vi "Dashboard Main.vi"() -> ()   [LabVIEW 2012]
uses:
  <vilib>/event_ctls.llb/eventvkey.ctl
  <vilib>/Utility/config.llb/Read Key (String).vi
  <vilib>/Utility/config.llb/Read Key (I32).vi
  <vilib>/Utility/config.llb/Write Key (String).vi
  <vilib>/Utility/config.llb/Write Key (I32).vi
  <vilib>/Utility/config.llb/NI_LVConfig.lvlib
panel:
  out "Battery Value":dbl(slide) scale=0.0..14.0 scale format="%#_2e"
  out "Battery":sgl(graph)
  in  "Camera Settings":T1={"Frate Rate"=30, "Compression"=30, "Size"=1} {"Frate Rate" scale=1.0..30.0; "Size" items=["640x480", "320x240", "160x120"]}
  out "Mode":T2(ring)=enum."Auto Disabled"
  out "Camera IP":string
  out "JS1 Z":dbl(slide) scale=-1.0..1.0 scale format="%#_2e"
  out "JS2 Z":dbl(slide) scale=-1.0..1.0 scale format="%#_2e"
  out "Joystick 1":cluster{"X":dbl, "Y":dbl}[](graph)
  out "Joystick 2":cluster{"X":dbl, "Y":dbl}[](graph)
  out "JS Buttons 1":T3
  out "JS Buttons 2":T3
  out "MotorSlide4":dbl(slide) scale=-1.0..1.0 scale format="%#_2e"
  out "MotorSlide3":dbl(slide) scale=-1.0..1.0 scale format="%#_2e"
  out "MotorSlide2":dbl(slide) scale=-1.0..1.0 scale format="%#_2e"
  in  "MotorName3":string="Front Left"
  in  "MotorName4":string="Front Right"
  in  "MotorName1":string="Rear Left"
  in  "MotorName2":string="Rear Right"
  out "MotorChart4":dbl(graph)
  out "MotorChart3":dbl(graph)
  out "MotorChart2":dbl(graph)
  out "MotorSlide1":dbl(slide) scale=-1.0..1.0 scale format="%#_2e"
  out "MotorChart1":dbl(graph)
  out "Robot IP":string
  in  "Dashboard Tab":enum32{"Operation", "Test", "Checklist"}(tab)
  in  "Checkbox 2":bool
  in  "Checkbox 1":bool
  in  "Slider 1":dbl(slide) scale=0.0..100.0
  out "array of clusters":cluster{"vi reference":refnum<vi>}[](array[cluster])
  in  "Slider":dbl(slide) scale=0.0..100.0 scale format="%#_3g"
  in  "On/Off":bool caption="Solenoid"
  in  "Test Name":u16(ring) items=["Select the test to run...", "Example Test", "-------------------------------", "List of tests is built in robot code.", "Replace with your own automated tests."]
  in  "Test Tree":string(tree)
  in  "Motor":cluster{"Value":dbl, "Enable":bool} {"Value" scale=-1.0..1.0 scale format="%#_3g"}
  out "Progress":T4 {"Test Progress" scale=0.0..100.0}
  in  "Rev/Fwd":cluster{"Forward":bool, "Reverse":bool}
  in  "Ring":u16(ring) items=["Auto", "Fixed indoor", "Fixed outdoor 1", "Fixed outdoor 2", "Fixed fluorescent 1", "Fixed fluorescent 2", "Hold current"]
  in  "Listbox":i32(listbox)
  in  "Viewer":T5(tab)
  out "Mbps":dbl format="%#.1g"
  in  "Enable":bool
  in  "DB Camera Config":bool
  out "Mbps":bool
  out "fps":dbl format="%#.1g"
  out "Image Error Message":string="Timeout in Camera Communications"
  out "Camera Image":T6(plugin-control)
  out "Buttons 1":cluster{"1":bool, "2":bool, "3":bool}
  out "Kinect 1":cluster{"X":dbl, "Y":dbl, "Z":dbl} {"X" scale=1.0..-1.0; "Y" scale=1.0..-1.0; "Z" scale=1.0..-1.0}
  out "Buttons 2":cluster{"1":bool, "2":bool, "3":bool}
  out "Kinect 2":cluster{"X":dbl, "Y":dbl, "Z":dbl} {"X" scale=1.0..-1.0; "Y" scale=1.0..-1.0; "Z" scale=1.0..-1.0}
  out "Version":string
  out "Skeleton Picture":picture
  out "Players":i8
  out "Tree":string(tree)
  # "Drive & Motors"
  # "Robot IP:"
  # "Customize by placing controls and indicators here and name to match\nDashboard Variables on robot."
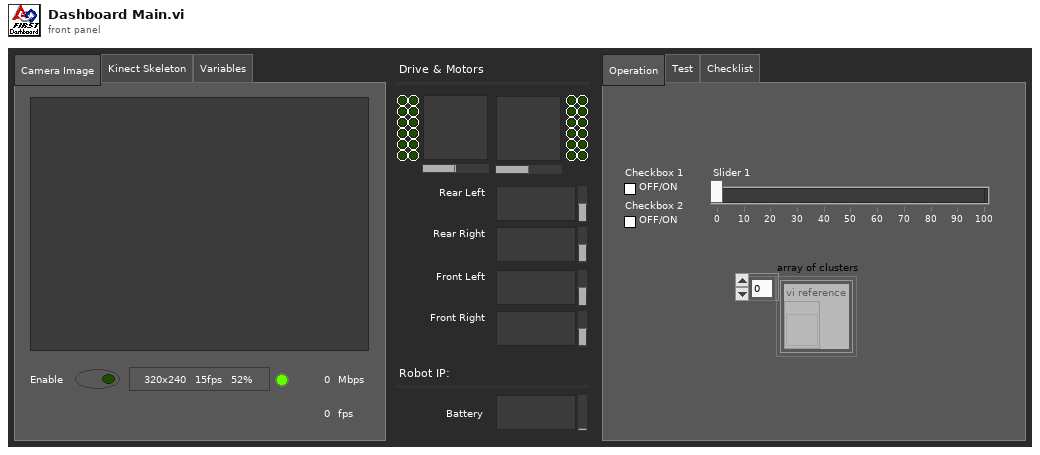
[diagram p1: front panel]
types:
  T1 = cluster{"Frate Rate":i32, "Compression":i32, "Size":u16}
  T2 = enum8{"Tele-Op Disabled", "Tele-Op Enabled", "Auto Disabled", "Auto Enabled", "Test Disabled", "Test Enabled", ""}
  T3 = cluster{bool, bool, bool, bool, bool, bool, bool, bool, bool, bool, bool, bool}
  T4 = cluster{"Test Progress":u8, "Test Progress Text":string}
  T5 = enum32{"Camera Image", "Kinect Skeleton", "Variables"}
  T6 = typedef "IMAQ Image.ctl" = refnum<image>
  T7 = typedef "Image Type" = u32
  T8 = typedef "LVBoundsTypeDef.ctl" = cluster{"Width":u32, "Height":u32}
  T9 = typedef "SkeletonTrackState.ctl" = enum32{"NotTracked", "PositionOnly", "Tracked"}
  T10 = cluster{"TrackingState":u8[], "Position":cluster{"x":sgl, "y":sgl, "z":sgl}, cluster{"x":sgl, "y":sgl, "z":sgl, sgl}[], "TrackState":T9}
  T11 = cluster{cluster{"ScaledToPercentRange":dbl, "ScaledToPercentRange":dbl, "ScaledToPercentRange":dbl}, cluster{bool, bool, bool}}[]
  T12 = cluster{cluster{"ScaledToPercentRange":dbl, "ScaledToPercentRange":dbl, "ScaledToPercentRange":dbl}, cluster{bool, bool, bool}}
  T13 = cluster{"ScaledToPercentRange":dbl, "ScaledToPercentRange":dbl, "ScaledToPercentRange":dbl}
  T14 = typedef "LVRectTypeDef.ctl" = cluster{"Left":i16, "Top":i16, "Right":i16, "Bottom":i16}
  T15 = cluster{"Competition mode":bool, "Robot Link":bool, "Autonomous":bool, "Enabled":bool, "E-Stop":bool, "Simulated":bool, "TestMode":bool, "Docked Window":bool}
  T16 = cluster{"Boolean Array[0]":bool, "Boolean Array[1]":bool, "Boolean Array[2]":bool, "Boolean Array[3]":bool, "Boolean Array[4]":bool, "Boolean Array[5]":bool, "Boolean Array[6]":bool, "Boolean Array[7]":bool, "Boolean Array[8]":bool, "Boolean Array[9]":bool, "Boolean Array[10]":bool, "Boolean Array[11]":bool}
  T17 = typedef "NI_LVConfig.lvlib/Config Data RefNum.ctl" = refnum<k1>
  T18 = typedef "eventvkey.ctl" = enum16{"ASCII", "Enter", "Return", "Shift", "Ctrl", "Alt", "Cmd", "Opt", "Caps", "NumLock", "Clear", "Break", "Up", "Down", "Left", "Right", "Insert", "Delete", "Home", "End", "PageUp", "PageDown", "Escape", "Help", "Pause", "ScrollLock", "F1", "F2", "F3", "F4", "F5", "F6", "F7", "F8", "F9", "F10", "F11", "F12", "F13", "F14", "F15", "F16", "F17", "F18", "F19", "F20", "F21", "F22", "F23", "F24", "Play", "VolumeUp", "VolumeDown", "Mute", "Two Byte Char"}
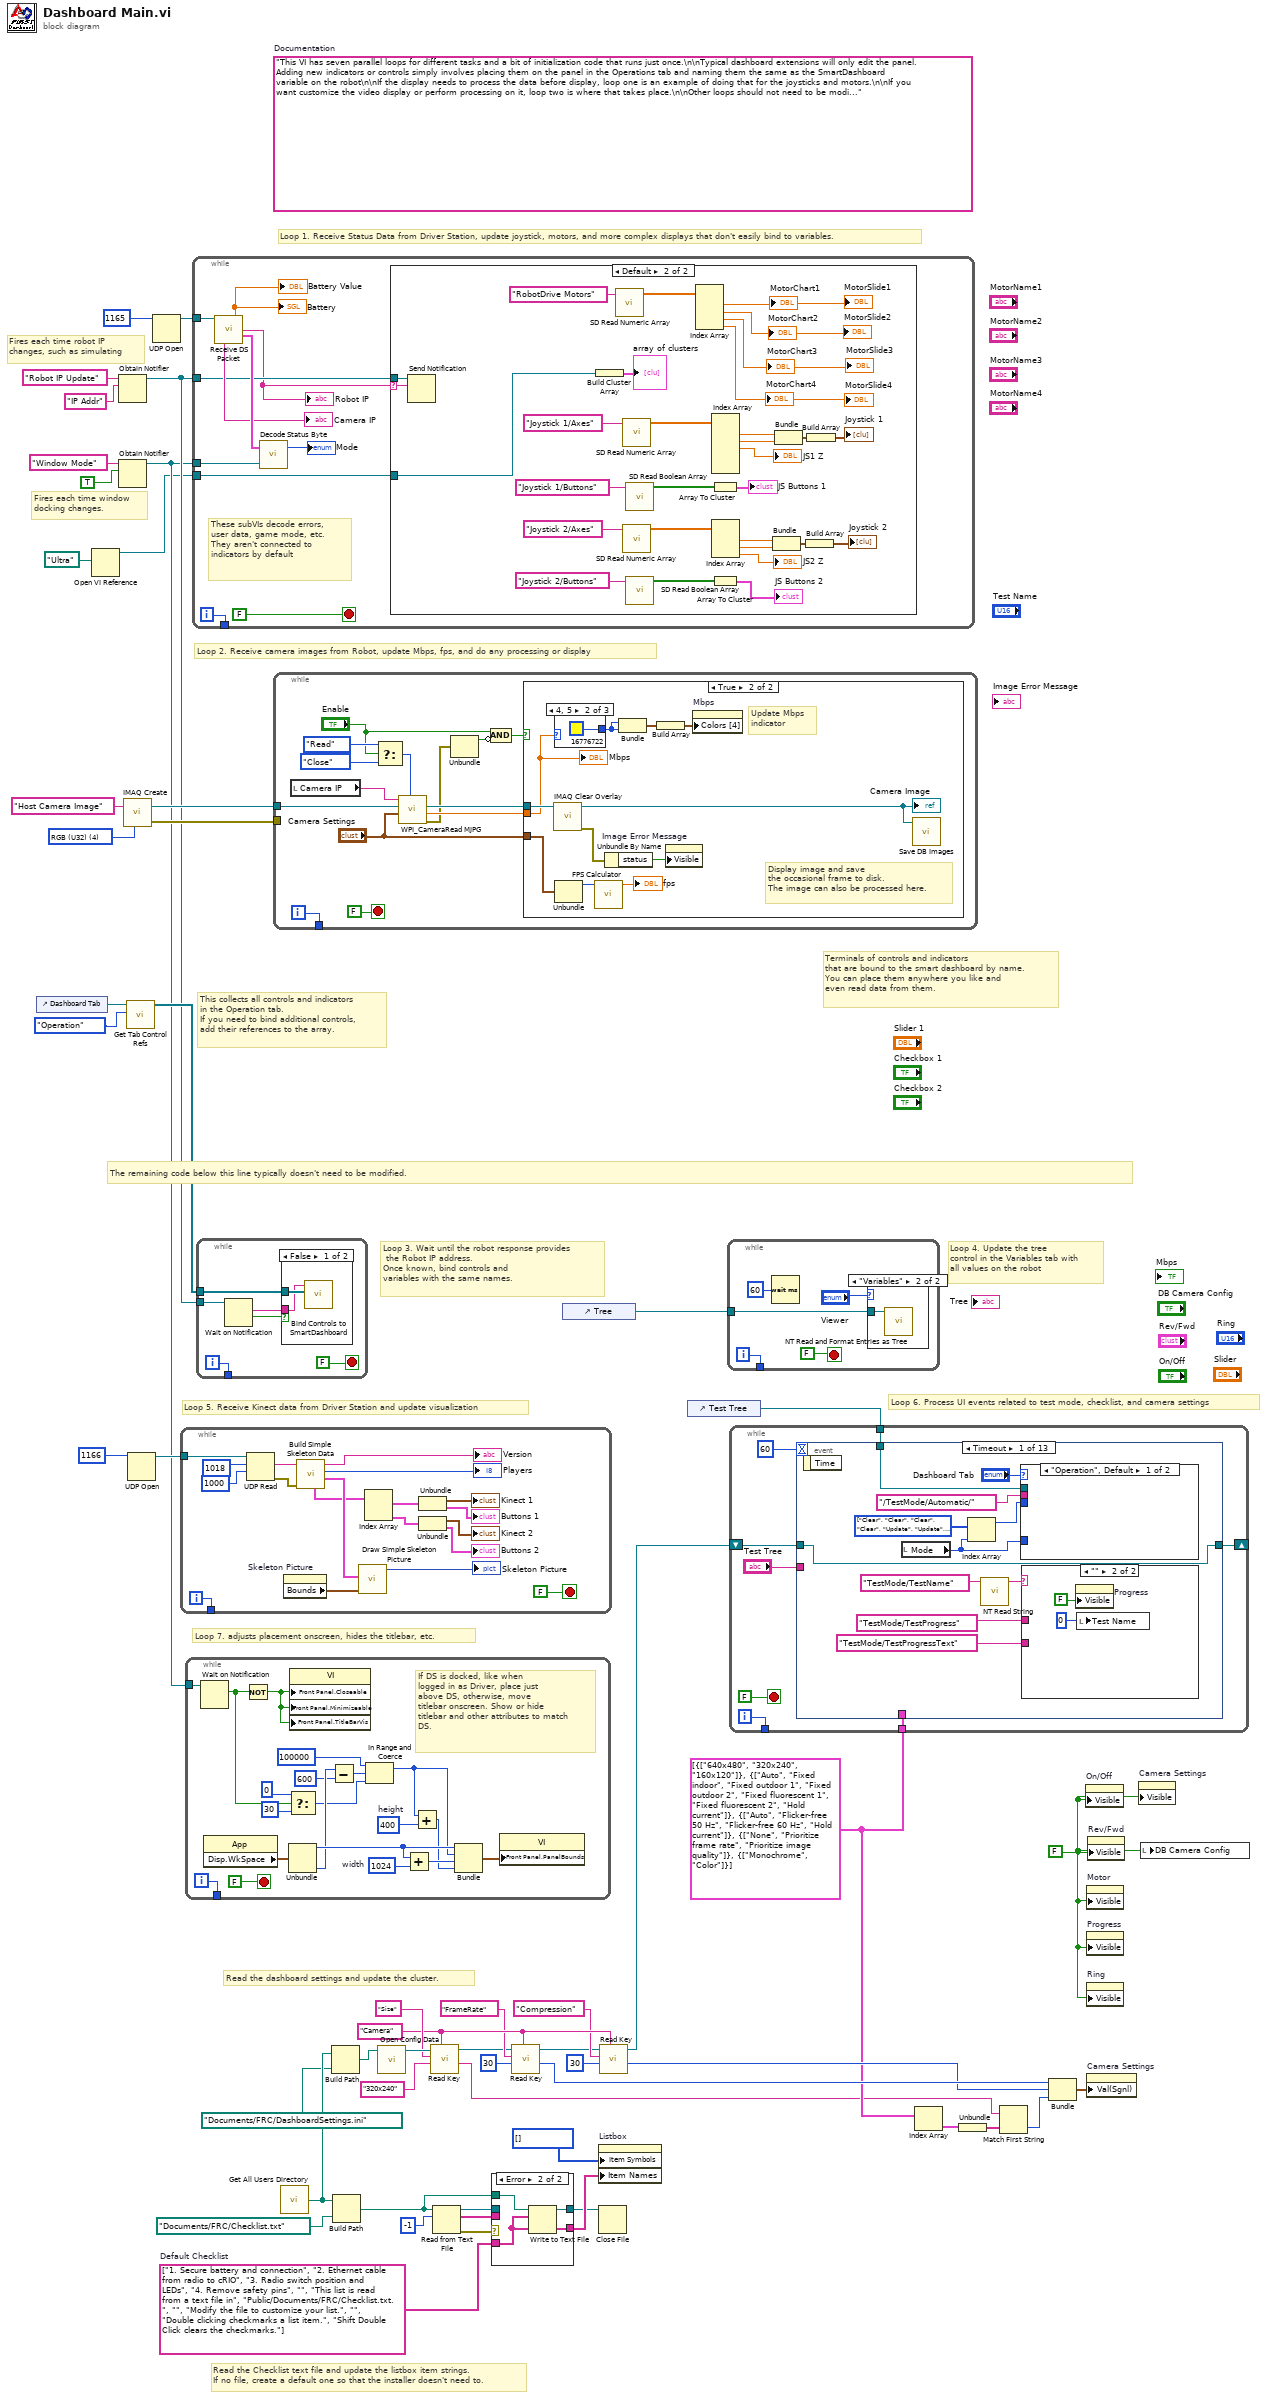
[diagram p0: block diagram]
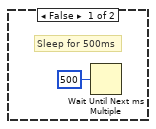
[diagram p3: hidden frame]
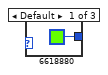
[diagram p4: hidden frame]
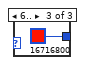
[diagram p5: hidden frame]
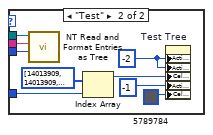
[diagram p7: hidden frame]
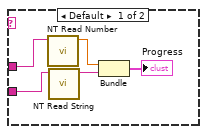
[diagram p8: hidden frame]
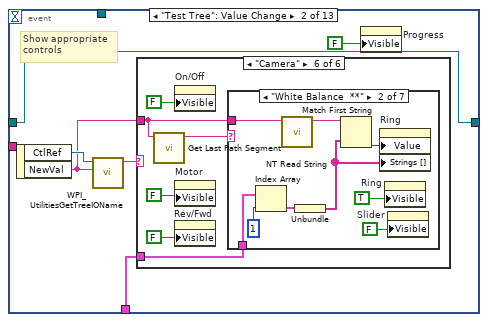
[diagram p9: hidden frame]
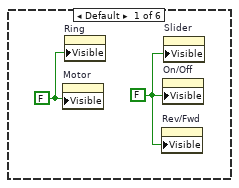
[diagram p10: hidden frame]
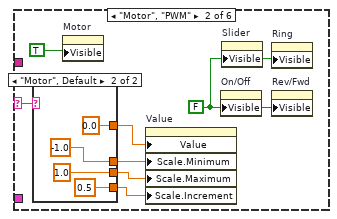
[diagram p11: hidden frame]
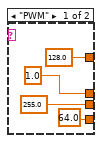
[diagram p12: hidden frame]
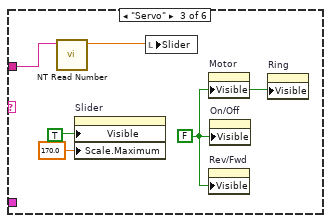
[diagram p13: hidden frame]
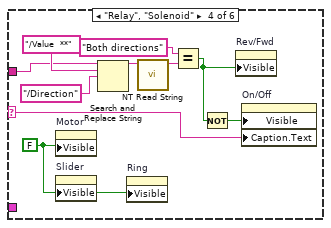
[diagram p14: hidden frame]
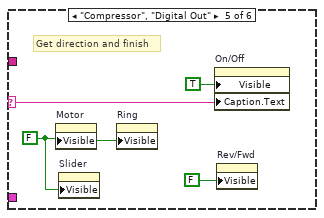
[diagram p15: hidden frame]
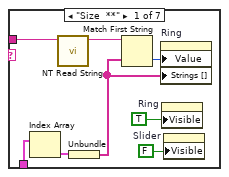
[diagram p16: hidden frame]
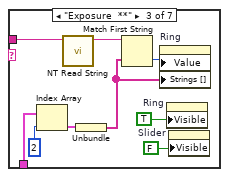
[diagram p17: hidden frame]
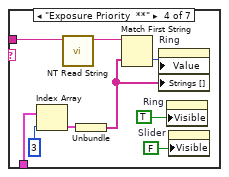
[diagram p18: hidden frame]
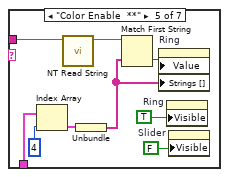
[diagram p19: hidden frame]
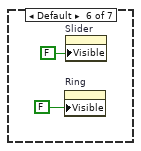
[diagram p20: hidden frame]
diagram:
  w23 = "Camera"
  w15 = cluster{string[]}[] [{["640x480", "320x240", "160x120"]}, {["Auto", "Fixed indoor", "Fixed outdoor 1", "Fixed outdoor 2", "Fixed fluorescent 1", "Fixed fluorescent 2", "Hold current"]}, {["Auto", "Flicker-free 50 Hz", "Flicker-free 60 Hz", "Hold current"]}, {["None", "Prioritize frame rate", "Prioritize image quality"]}, {["Monochrome", "Color"]}]
  w31 = string[] ["1. Secure battery and connection", "2. Ethernet cable from radio to cRIO", "3. Radio switch position and LEDs", "4. Remove safety pins", "", "This list is read from a text file in", "Public/Documents/FRC/Checklist.txt.", "", "Modify the file to customize your list.", "", "Double clicking checkmarks a list item.", "Shift Double Click clears the checkmarks."]  # Default Checklist
  w29 = FALSE ("Visible")
  (unwired) "This VI has seven parallel loops for different tasks and a bit of initialization code that runs just once.\n\nTypical dashboard extensions will only edit the panel. Adding new indicators or controls simply involves placing them on the panel in the Operations tab and naming them the same as the SmartDashboard variable on the robot\n\nIf the display needs to process the data before display, loop one is an example of doing that for the joysticks and motors.\n\nIf you want customize the video display or perform processing on it, loop two is where that takes place.\n\nOther loops should not need to be modified. They are pretty standard, and document the task they perform."  # Documentation
  w52 = T7 4 items=["Grayscale (U8)", "Grayscale (I16)", "Grayscale (SGL)", "Complex (CSG)", "RGB (U32)", "HSL (U32)", "RGB (U64)"] ("Image Type")
  # "Fires each time robot IP\nchanges, such as simulating"
  # "Fires each time window\ndocking changes."
  # "Read the Checklist text file and update the listbox item strings.\nIf no file, create a default one so that the installer doesn't need to."
  # "This collects all controls and indicators\nin the Operation tab.\nIf you need to bind additional controls,\nadd their references to the array."
  # "The remaining code below this line typically doesn't need to be modified."
  # "Loop 6. Process UI events related to test mode, checklist, and camera settings"
  # "Read the dashboard settings and update the cluster."
  # "Terminals of controls and indicators\nthat are bound to the smart dashboard by name.\nYou can place them anywhere you like and\neven read data from them."
  # "Loop 4. Update the tree\ncontrol in the Variables tab with\nall values on the robot"
  # "Loop 3. Wait until the robot response provides\n the Robot IP address.\nOnce known, bind controls and\nvariables with the same names."
  # "Loop 5. Receive Kinect data from Driver Station and update visualization"
  # "Loop 7. adjusts placement onscreen, hides the titlebar, etc."
  # "Loop 1. Receive Status Data from Driver Station, update joystick, motors, and more complex displays that don't easily bind to variables."
  # "Loop 2. Receive camera images from Robot, update Mbps, fps, and do any processing or display"
  n1 = control-ref of="Dashboard Tab"() -> (w45:refnum<vi>)
  n2 = Open VI Reference(vi path=path "Ultra") -> (vi reference=w1:refnum<vi>)  [unwired: 5 in, 1 out]
  n3 = Obtain Notifier(name (unnamed)="Robot IP Update", notification data type="IP Addr" ("name (unnamed)")) -> (notifier out=w42:refnum<notifier>)  [unwired: 2 in, 2 out]
  n4 = Obtain Notifier(name (unnamed)="Window Mode", notification data type=TRUE) -> (notifier out=w35:refnum<notifier>)  [unwired: 2 in, 2 out]
  n5 = call "IMAQ Create"("Image Name"="Host Camera Image", "Image Type"=w52) -> ("New Image"=w50:T6, "error out"=w49:errorcluster)  [unwired: 2 in, 1 out]
  n6 = call <vilib>:"Get Tab Control Refs.vi"("Page Index"=enum32{"Operation", "Test"}."Operation" ("Dashboard Tab"), "TabControl in"=w45) -> ("ControlsOnPage"=w46:refnum<vi>[])  [unwired: 9 in]
  n7 = UDP Open(11:u16 1166 ("port")) -> (port=w47:refnum<k16>)  [unwired: 2 in, 4 out]
  n8 = UDP Open(11:u16 1165 ("port")) -> (port=w53:refnum<k16>)  [unwired: 2 in, 4 out]
  n9 = while {
    tunnel: w47 -> [w71]
    tunnel: [w56] -> _
    i -> [w56]
    stop <- FALSE stop-if-true
    n10 = UDP Read(connection ID=w71, max size (548)=1018 ("bytes to read"), timeout ms (25000)=1000) -> (data out=w65:string, error out=w55:errorcluster)  [unwired: 1 in, 3 out]
    n11 = property on="Skeleton Picture" class="Pict"() -> ("Bounds"=w67:T8)  [unwired: 2 in, 2 out]
    n12 = call "Build Simple Skeleton Data.vi"("error in (no error)"=w55, "data in"=w65) -> ("Skeleton Data"=w66:T10, "NumPlayers"=→"Players":i8, "Version String"=→"Version":string, "Simple Joystick Info"=w63:T11)  [unwired: 5 in, 1 out]
    n13 = call "Draw Simple Skeleton Picture.vi"("Bounds"=w67, "Simple Skeleton"=w66) -> ("new picture out"=→"Skeleton Picture":picture)  [unwired: 9 in]
    n14 = Index Array(array=w63) -> (element #1=w62:T12, element #2=w61:T12)  [unwired: 2 in]
    n15 = Unbundle(w62) -> (→"Kinect 1":T13, →"Buttons 1":cluster{bool, bool, bool})
    n16 = Unbundle(w61) -> (→"Kinect 2":T13, →"Buttons 2":cluster{bool, bool, bool})
  }
  n17 = while {
    tunnel: w35 -> [w92]
    tunnel: [w90] -> _
    i -> [w90]
    stop <- FALSE stop-if-true
    w82 = 1024  # width
    w85 = 400  # height
    # "If DS is docked, like when\nlogged in as Driver, place just\nabove DS, otherwise, move\ntitlebar onscreen. Show or hide\ntitlebar and other attributes to match\nDS."
    n18 = Wait on Notification(notifier=w92) -> (notification=w77:bool)  [unwired: 3 in, 3 out]
    n19 = property class="App"() -> ("Disp.WkSpace"=w88:T14)  [unwired: 2 in, 2 out]
    n20 = Not(x=w77) -> (.not. x?=w91:bool)
    n21 = Unbundle(w88) -> ("Left"=w86:i16, "Bottom"=w83:i16)  [unwired: 2 out]
    n22 = Select(t=0, s=w77, f=30) -> (s? t:f=w76:i32)
    n23 = property class="VI"("Front Panel.Closeable"=w91, "Front Panel.Minimizeable"=w91, "Front Panel.TitleBarVis"=w91) -> ()  [unwired: 2 in, 2 out]
    n24 = Subtract(x=w83, y=600) -> (x-y=w80:i32)
    n25 = In Range and Coerce(upper limit=100000, x=w80, lower limit=w76) -> (coerced(x)=w74:i32)  [unwired: 1 out]
    n26 = Add(x=w86, y=w82) -> (x+y=w87:i32)
    n27 = Add(x=w74, y=w85) -> (x+y=w84:i32)
    n28 = Bundle("Left"=w86, w74, w87, w84) -> (w89:cluster{"Left":i16, i32, i32, i32})  [unwired: 1 out]
    n29 = property class="VI"("Front Panel.PanelBounds"=w89) -> ()  [unwired: 2 in, 2 out]
  }
  n30 = while {
    tunnel: w53 -> [w102]
    tunnel: w42 -> [w96]
    tunnel: w35 -> [w100]
    tunnel: [w97] -> _
    tunnel: w1 -> [w94]
    i -> [w97]
    stop <- FALSE stop-if-true
    # "These subVIs decode errors, user data, game mode, etc.\nThey aren't connected to indicators by default"
    n31 = call "Receive DS Packet.vi"("Recv Socket"=w102) -> ("Battery"=→"Battery" →"Battery Value":sgl, "Robot IP Address"=w95:string, "Status"=w103:T15, "Camera IP Address"=→"Camera IP":string)  [unwired: 1 in, 10 out]
    "Robot IP" <- w95
    n32 = call "Decode Status Byte.vi"("Window Mode Notifier"=w100, "Status"=w103) -> ("Mode"=→"Mode":T2)  [unwired: 1 out]
    n33 = case shown="Default" w95 {
      selector: w95 -> [_ w107]
      tunnel: w96 -> [_ w108]
      tunnel: w94 -> [_ w105]
      frame "0.0.0.0" {
        # "Robot not responding, don't poll the variables"
      }
      frame Default {
        n34 = Send Notification(notification=w107, notifier=w108) -> ()  [unwired: 1 in, 2 out]
        n35 = Build Cluster Array(w105) -> (→"array of clusters":cluster{"vi reference":refnum<vi>}[])
        n36 = call <vilib>:"SD Read Numeric Array.vi"("Name"="RobotDrive Motors") -> ("Numeric Array"=w131:dbl[])  [unwired: 8 in, 2 out]
        n37 = call <vilib>:"SD Read Numeric Array.vi"("Name"="Joystick 1/Axes") -> ("Numeric Array"=w124:dbl[])  [unwired: 8 in, 2 out]
        n38 = call <vilib>:"SD Read Numeric Array.vi"("Name"="Joystick 2/Axes") -> ("Numeric Array"=w118:dbl[])  [unwired: 8 in, 2 out]
        n39 = call <vilib>:"SD Read Boolean Array.vi"("Name"="Joystick 1/Buttons") -> ("Boolean Array"=w126:bool[])  [unwired: 8 in, 2 out]
        n40 = call <vilib>:"SD Read Boolean Array.vi"("Name"="Joystick 2/Buttons") -> ("Boolean Array"=w117:bool[])  [unwired: 8 in, 2 out]
        n41 = Index Array(array=w131) -> (element #1=→"MotorChart1" →"MotorSlide1":dbl, element #2=→"MotorSlide2" →"MotorChart2":dbl, element #3=→"MotorChart3" →"MotorSlide3":dbl, element #4=→"MotorChart4" →"MotorSlide4":dbl)  [unwired: 4 in]
        n42 = Array To Cluster(array=w126) -> (cluster=→"JS Buttons 1":T16)
        n43 = Array To Cluster(array=w117) -> (cluster=→"JS Buttons 2":T16)
        n44 = Index Array(array=w124) -> (element #1=w121:dbl, element #2=w122:dbl, element #3=→"JS1 Z":dbl)  [unwired: 6 in, 3 out]
        n45 = Index Array(array=w118) -> (element #1=w113:dbl, element #2=w112:dbl, element #3=→"JS2 Z":dbl)  [unwired: 3 in]
        n46 = Bundle("Numeric"=w113, "Numeric"=w112) -> (w114:cluster{"Numeric":dbl, "Numeric":dbl})  [unwired: 1 in]
        n47 = Bundle("Numeric"=w121, "Numeric"=w122) -> (w120:cluster{"Numeric":dbl, "Numeric":dbl})  [unwired: 1 in]
        n48 = Build Array(w114) -> (→"Joystick 2":cluster{"Numeric":dbl, "Numeric":dbl}[])
        n49 = Build Array(w120) -> (→"Joystick 1":cluster{"Numeric":dbl, "Numeric":dbl}[])
      }
    }
  }
  n50 = while {
    tunnel: w46 -> [w140]
    tunnel: w42 -> [w137]
    tunnel: [w135] -> _
    i -> [w135]
    stop <- FALSE stop-if-true
    n51 = Wait on Notification(notifier=w137) -> (notification=w136:string, timed out?=w138:bool)  [unwired: 3 in, 2 out]
    n52 = case shown="False" w138 {
      tunnel: w140 -> [w142 _]
      tunnel: w136 -> [w141 _]
      frame False {
        n53 = call <vilib>:"Bind Controls to SmartDashboard.vi"("Bound Control Refs"=w142, "Server IP Address"=w141) -> ()  [unwired: 10 in]
      }
      frame True {
      }
    }
  }
  n54 = while {
    tunnel: w50 -> [w152]
    tunnel: w49 -> [_]
    tunnel: [w155] -> _
    i -> [w155]
    stop <- FALSE stop-if-true
    n55 = local read "Camera IP"() -> (w154:string)
    n56 = Select(t=enum16{"Read", "Reopen", "Close"}."Read" ("Operation"), s="Enable", f=enum16{"Read", "Reopen", "Close"}."Close" ("Operation")) -> (s? t:f=w147:enum16{"Read", "Reopen", "Close"})
    n57 = call <vilib>:"WPI_CameraRead MJPG.vi"("Operation"=w147, "Camera Settings"="Camera Settings", "Image"=w152, "address"=w154) -> ("error out"=w146:errorcluster, "Bandwidth (kbps)"=w150:dbl, "Image Out"=w151:T6)  [unwired: 5 in]
    n58 = Unbundle(w146) -> ("status"=w144:bool)  [unwired: 2 out]
    n59 = Compound Arithmetic op=AND("Enable", invert w144) -> (w143:bool)
    n60 = case shown="True" w143 {
      tunnel: "Camera Settings" -> [_ w159]
      tunnel: w151 -> [_ w162]
      tunnel: w150 -> [_ w161]
      frame False {
        # "Sleep for 500ms"
        n61 = Wait Until Next ms Multiple(millisecond multiple=u32 500) -> ()  [unwired: 1 out]
      }
      frame True {
        # "Display image and save\nthe occasional frame to disk.\nThe image can also be processed here."
        # "Update Mbps\nindicator"
        n62 = call "IMAQ Clear Overlay"("Image"=w162) -> ("error out"=w167:errorcluster, "Image Out"=w166:T6)  [unwired: 2 in, 7 out]
        "Camera Image" <- w166
        n63 = case shown="4, 5" w161 {
          tunnel: [u32 6618880 ("Color Box") u32 16776722 ("Color Box") u32 16716800 ("Color Box")] -> w163
          frame Default {
          }
          frame 4, 5 {
          }
          frame 6.. {
          }
        }
        n64 = Unbundle(w159) -> ("Frate Rate"=w158:i32)  [unwired: 2 out]
        n65 = call "FPS Calculator.vi"("Average Count"=w158) -> ("fps"=→"fps":dbl)  [unwired: 10 in]
        n66 = Unbundle By Name(w167) -> ("status"=w168:bool)
        n67 = Bundle("Color Box"=w163, "Color Box"=w163) -> (w165:cluster{"Color Box":u32, "Color Box":u32})  [unwired: 1 out]
        n68 = Build Array(w165) -> (w164:cluster{"Color Box":u32, "Color Box":u32}[])
        n69 = property on="Image Error Message" class="Str"("Visible"=w168) -> ()  [unwired: 2 in, 2 out]
        n70 = property on="Mbps" class="Bool (strict)"("Colors [4]"=w164) -> ()  [unwired: 2 in, 2 out]
        n71 = call "Save DB Images.vi"("Image"=w166) -> ()  [unwired: 2 in, 1 out]
        "Mbps" <- w161
      }
    }
  }
  n72 = call "Get All Users Directory.vi"() -> ("All User Path"=w28:path)
  n73 = Build Path(base path=w28, name or relative path=path "Documents/FRC/DashboardSettings.ini") -> (appended path=w27:path)
  n74 = Build Path(base path=w28, name or relative path=path "Documents/FRC/Checklist.txt") -> (appended path=w32:path)
  n75 = call <vilib>:"Open Config Data.vi"("configuration file path"=w27) -> ("refnum"=w26:T17)  [unwired: 8 in, 2 out]
  n76 = call-poly <vilib>:"Read Key.vi"("section"=w23, "default value"="320x240", "key"="Size", "refnum"=w26) -> ("value"=w13:string, "refnum out"=w8:T17)  [unwired: 2 in, 4 out]
  n77 = Read from Text File(file (use dialog)=w32, count=-1 ("timeout ms (25000)")) -> (refnum out=w10:refnum<file>, text=w33:string[], error out=w34:errorcluster)  [unwired: 2 in, 1 out]
  n78 = case shown="Error" w34 {
    tunnel: w33 -> [w173 _]
    tunnel: [w173 w175] -> w30
    tunnel: w31 -> [_ w175]
    tunnel: w32 -> [_ w176]
    tunnel: [w172 w174] -> w9
    tunnel: w10 -> [w172 _]
    frame No Error {
    }
    frame Error {
      n79 = Write to Text File(file (use dialog)=w176, text=w175) -> (refnum out=w174:refnum<file>)  [unwired: 2 in, 2 out]
    }
  }
  n80 = call-poly <vilib>:"Read Key.vi"("section"=w23, "default value"=30, "key"="FrameRate", "refnum"=w8) -> ("value"=w18:i32, "refnum out"=w7:T17)  [unwired: 1 in, 5 out]
  n81 = control-ref of="Tree"() -> (w4:refnum<vi>)
  n82 = property on="Listbox" class="LstBox (strict)"("Item Symbols"=i32[] [], "Item Names"=w30) -> ()  [unwired: 2 in, 2 out]
  n83 = Close File(refnum=w9) -> ()  [unwired: 1 in, 2 out]
  n84 = call-poly <vilib>:"Read Key.vi"("section"=w23, "default value"=30, "key"="Compression", "refnum"=w7) -> ("value"=w17:i32, "refnum out"=w5:T17)  [unwired: 1 in, 5 out]
  n85 = control-ref of="Test Tree"() -> (w3:refnum<vi>)
  n86 = while {
    tunnel: [w178] -> _
    tunnel: w4 -> [w177]
    i -> [w178]
    stop <- FALSE stop-if-true
    n87 = Wait (ms)(milliseconds to wait=u32 60) -> ()  [unwired: 1 out]
    n88 = case shown="\"Variables\"" "Viewer" {
      tunnel: w177 -> [_ w182]
      frame Default {
      }
      frame "Variables" {
        n89 = call <vilib>:"NT Read and Format Entries as Tree.vi"("Tree Refnum"=w182) -> ()  [unwired: 9 in, 2 out]
      }
    }
  }
  n90 = while {
    tunnel: w15 -> [w187]
    shift-right: [w186] -> _
    shift-left: w5 -> [w185]
    tunnel: [w184] -> _
    tunnel: w3 -> [w183]
    i -> [w184]
    stop <- FALSE stop-if-true
    n91 = event shown="[0] Timeout" {
      selector: _ -> [_ _ _ _ _ _ _ _ _ _ _ _ _]
      dyn-events: _ -> [_ _ _ _ _ _ _ _ _ _ _ _ _]
      timeout: u32 60 ("milliseconds to wait") -> [_ _ _ _ _ _ _ _ _ _ _ _ _]
      tunnel: w183 -> [w197 _ _ _ _ _ _ _ _ _ _ _ _]
      tunnel: "Test Tree" -> [_ _ _ _ _ _ _ _ w391 w399 w401 w405 w413]
      tunnel: w187 -> [_ w219 _ _ _ _ w355 w385 _ _ _ _ _]
      tunnel: [w191 w218 _ w321 w329 w341 w354 w378 w390 w397 w400 w404 w412] -> w186
      tunnel: w185 -> [w191 w218 _ w321 w329 w341 w353 w378 w390 w397 w400 w404 w412]
      event Timeout {
        w196 = enum16{"Update", "Clear"}[] [enum."Clear", enum."Clear", enum."Clear", enum."Clear", enum."Update", enum."Update", enum."Clear"] items=["Update", "Clear"]
        n92 = event-data() -> ()  [unwired: 1 in, 1 out]
        n93 = local read "Mode"() -> (w194:T2)
        n94 = Index Array(array=w196, index=w194) -> (element=w195:enum16{"Update", "Clear"})
        n95 = call <vilib>:"NT Read String.vi"("Name"="TestMode/TestName") -> ("String"=w200:string)  [unwired: 9 in, 1 out]
        n96 = case shown="\"Operation\", Default" "Dashboard Tab" {
          tunnel: w197 -> [_ w210]
          tunnel: "/TestMode/Automatic/" ("Name Pattern") -> [_ w209]
          tunnel: w195 -> [_ w208]
          tunnel: w194 -> [_ w206]
          frame "Operation", Default {
          }
          frame "Test" {
            w205 = -2 ("Active Item:Row Number")
            n97 = call <vilib>:"NT Read and Format Entries as Tree.vi"("Operation"=w208, "Name Pattern"=w209, "Tree Refnum"=w210) -> ()  [unwired: 7 in, 2 out]
            n98 = Index Array(array=u32[] [14013909, 14013909, 14013909, 14013909, 14013909, 16777215, 14013909], index=w206) -> (element=w204:u32)
            n99 = property on="Test Tree" class="Tree (strict)"("Active Item Row Number"=w205, "ActiveColNum"=w205, "CellBG"=w204, "Active Item Row Number"=-1 ("Active Item:Row Number"), "CellBG"=u32 5789784 ("Color Box")) -> ()  [unwired: 2 in, 2 out]
          }
        }
        n100 = case shown="\"\"" w200 {
          tunnel: "TestMode/TestProgress" ("Name") -> [w212 _]
          tunnel: "TestMode/TestProgressText" ("Name") -> [w211 _]
          frame Default {
            n101 = call <vilib>:"NT Read Number.vi"("Name"=w212) -> ("Numeric"=w213:dbl)  [unwired: 9 in, 1 out]
            n102 = call <vilib>:"NT Read String.vi"("Name"=w211) -> ("String"=w214:string)  [unwired: 9 in, 1 out]
            n103 = Bundle("Numeric"=w213, "String"=w214) -> (→"Progress":cluster{"Numeric":dbl, "String":string})  [unwired: 1 in]
          }
          frame "" {
            n104 = property on="Progress" class="Clust (strict)"("Visible"=FALSE) -> ()  [unwired: 2 in, 2 out]
            n105 = local write "Test Name"(u16 0) -> ()
          }
        }
      }
      event "Test Tree": Value Change {
        # "Show appropriate\ncontrols"
        n106 = event-data() -> ("CtlRef"=w222:refnum<vi>, "NewVal"=w220:string)  [unwired: 1 in]
        n107 = call <vilib>:"WPI_UtilitiesGetTreeIOName.vi"("NewVal"=w220, "TreeControl in"=w222) -> ("I/O Name"=w223:string)  [unwired: 9 in]
        n108 = case shown="\"Camera\"" w223 {
          selector: w223 -> [_ w230 _ w248 w257 _]
          tunnel: w220 -> [_ _ w245 w247 _ w264]
          tunnel: w219 -> [_ _ _ _ _ w263]
          frame Default {
            w225 = FALSE ("Visible")
            w224 = FALSE ("Visible")
            n109 = property on="Motor" class="Clust (strict)"("Visible"=w224) -> ()  [unwired: 2 in, 2 out]
            n110 = property on="Ring" class="Ring (strict)"("Visible"=w224) -> ()  [unwired: 2 in, 2 out]
            n111 = property on="Rev/Fwd" class="Clust (strict)"("Visible"=w225) -> ()  [unwired: 2 in, 2 out]
            n112 = property on="On/Off" class="Bool (strict)"("Visible"=w225) -> ()  [unwired: 2 in, 2 out]
            n113 = property on="Slider" class="Slide (strict)"("Visible"=w225) -> ()  [unwired: 2 in, 2 out]
          }
          frame "Motor", "PWM" {
            w231 = FALSE ("Visible")
            n114 = case shown="\"Motor\", Default" w230 {
              tunnel: [1.0 ("Value") -1.0 ("Value")] -> w229
              tunnel: [255.0 ("Value") 1.0 ("Value")] -> w228
              tunnel: [128.0 ("Value") 0.0 ("Value")] -> w227
              tunnel: [64.0 ("Value") 0.5 ("Value")] -> w226
              frame "PWM" {
              }
              frame "Motor", Default {
              }
            }
            n115 = property on="Motor" class="Clust (strict)"("Visible"=TRUE) -> ()  [unwired: 2 in, 2 out]
            n116 = property on="Value" class="Slide (strict)"("Value"=w227, "Scale.Minimum"=w229, "Scale.Maximum"=w228, "Scale.Increment"=w226) -> ()  [unwired: 2 in, 2 out]
            n117 = property on="On/Off" class="Bool (strict)"("Visible"=w231) -> ()  [unwired: 2 in, 2 out]
            n118 = property on="Slider" class="Slide (strict)"("Visible"=w231) -> ()  [unwired: 2 in, 2 out]
            n119 = property on="Ring" class="Ring (strict)"("Visible"=w231) -> ()  [unwired: 2 in, 2 out]
            n120 = property on="Rev/Fwd" class="Clust (strict)"("Visible"=w231) -> ()  [unwired: 2 in, 2 out]
          }
          frame "Servo" {
            w243 = FALSE ("Visible")
            n121 = call <vilib>:"NT Read Number.vi"("Name"=w245) -> ("Numeric"=w244:dbl)  [unwired: 9 in, 1 out]
            n122 = property on="Slider" class="Slide (strict)"("Visible"=TRUE, "Scale.Maximum"=170.0 ("Scale.Range:Maximum")) -> ()  [unwired: 2 in, 2 out]
            n123 = local write "Slider"(w244) -> ()
            n124 = property on="Motor" class="Clust (strict)"("Visible"=w243) -> ()  [unwired: 2 in, 2 out]
            n125 = property on="Rev/Fwd" class="Clust (strict)"("Visible"=w243) -> ()  [unwired: 2 in, 2 out]
            n126 = property on="On/Off" class="Bool (strict)"("Visible"=w243) -> ()  [unwired: 2 in, 2 out]
            n127 = property on="Ring" class="Ring (strict)"("Visible"=w243) -> ()  [unwired: 2 in, 2 out]
          }
          frame "Relay", "Solenoid" {
            w246 = FALSE ("Visible")
            n128 = property on="Motor" class="Clust (strict)"("Visible"=w246) -> ()  [unwired: 2 in, 2 out]
            n129 = property on="Slider" class="Slide (strict)"("Visible"=w246) -> ()  [unwired: 2 in, 2 out]
            n130 = Search and Replace String(input string=w247, search string="/Value  **", replace string="/Direction") -> (result string=w253:string)  [unwired: 5 in, 3 out]
            n131 = property on="Ring" class="Ring (strict)"("Visible"=w246) -> ()  [unwired: 2 in, 2 out]
            n132 = call <vilib>:"NT Read String.vi"("Name"=w253) -> ("String"=w251:string)  [unwired: 9 in, 1 out]
            n133 = Equal?(x="Both directions", y=w251) -> (x = y?=w249:bool)
            n134 = Not(x=w249) -> (.not. x?=w250:bool)
            n135 = property on="Rev/Fwd" class="Clust (strict)"("Visible"=w249) -> ()  [unwired: 2 in, 2 out]
            n136 = property on="On/Off" class="Bool (strict)"("Visible"=w250, "Caption.Text"=w248) -> ()  [unwired: 2 in, 2 out]
          }
          frame "Compressor", "Digital Out" {
            w256 = FALSE ("Visible")
            # "Get direction and finish"
            n137 = property on="Motor" class="Clust (strict)"("Visible"=w256) -> ()  [unwired: 2 in, 2 out]
            n138 = property on="Slider" class="Slide (strict)"("Visible"=w256) -> ()  [unwired: 2 in, 2 out]
            n139 = property on="Ring" class="Ring (strict)"("Visible"=w256) -> ()  [unwired: 2 in, 2 out]
            n140 = property on="On/Off" class="Bool (strict)"("Visible"=TRUE, "Caption.Text"=w257) -> ()  [unwired: 2 in, 2 out]
            n141 = property on="Rev/Fwd" class="Clust (strict)"("Visible"=FALSE) -> ()  [unwired: 2 in, 2 out]
          }
          frame "Camera" {
            n142 = call <vilib>:"Get Last Path Segment.vi"("String in"=w264) -> ("String out"=w265:string)  [unwired: 10 in]
            n143 = property on="On/Off" class="Bool (strict)"("Visible"=FALSE) -> ()  [unwired: 2 in, 2 out]
            n144 = property on="Motor" class="Clust (strict)"("Visible"=FALSE) -> ()  [unwired: 2 in, 2 out]
            n145 = property on="Rev/Fwd" class="Clust (strict)"("Visible"=FALSE) -> ()  [unwired: 2 in, 2 out]
            n146 = case shown="\"White Balance  **\"" w265 {
              tunnel: w264 -> [w271 w280 w289 w298 w307 _ w313]
              tunnel: w263 -> [w269 w277 w286 w295 w304 _ _]
              frame "Size  **" {
                n147 = Index Array(array=w269) -> (element=w268:cluster{string[]})  [unwired: 1 in]
                n148 = call <vilib>:"NT Read String.vi"("Name"=w271) -> ("String"=w270:string)  [unwired: 9 in, 1 out]
                n149 = Unbundle(w268) -> (w266:string[])
                n150 = Match First String(2:w266, 3:w270) -> (0:w267:i32)  [unwired: 1 out]
                n151 = property on="Ring" class="Ring (strict)"("Value"=w267, "Strings []"=w266) -> ()  [unwired: 2 in, 2 out]
                n152 = property on="Ring" class="Ring (strict)"("Visible"=TRUE) -> ()  [unwired: 2 in, 2 out]
                n153 = property on="Slider" class="Slide (strict)"("Visible"=FALSE) -> ()  [unwired: 2 in, 2 out]
              }
              frame "White Balance  **" {
                n154 = Index Array(array=w277, index=1) -> (element=w278:cluster{string[]})
                n155 = call <vilib>:"NT Read String.vi"("Name"=w280) -> ("String"=w279:string)  [unwired: 9 in, 1 out]
                n156 = Unbundle(w278) -> (w275:string[])
                n157 = Match First String(2:w275, 3:w279) -> (0:w274:i32)  [unwired: 1 out]
                n158 = property on="Ring" class="Ring (strict)"("Value"=w274, "Strings []"=w275) -> ()  [unwired: 2 in, 2 out]
                n159 = property on="Ring" class="Ring (strict)"("Visible"=TRUE) -> ()  [unwired: 2 in, 2 out]
                n160 = property on="Slider" class="Slide (strict)"("Visible"=FALSE) -> ()  [unwired: 2 in, 2 out]
              }
              frame "Exposure  **" {
                n161 = Index Array(array=w286, index=2) -> (element=w287:cluster{string[]})
                n162 = call <vilib>:"NT Read String.vi"("Name"=w289) -> ("String"=w288:string)  [unwired: 9 in, 1 out]
                n163 = Unbundle(w287) -> (w283:string[])
                n164 = Match First String(2:w283, 3:w288) -> (0:w284:i32)  [unwired: 1 out]
                n165 = property on="Ring" class="Ring (strict)"("Value"=w284, "Strings []"=w283) -> ()  [unwired: 2 in, 2 out]
                n166 = property on="Ring" class="Ring (strict)"("Visible"=TRUE) -> ()  [unwired: 2 in, 2 out]
                n167 = property on="Slider" class="Slide (strict)"("Visible"=FALSE) -> ()  [unwired: 2 in, 2 out]
              }
              frame "Exposure Priority  **" {
                n168 = Index Array(array=w295, index=3) -> (element=w296:cluster{string[]})
                n169 = call <vilib>:"NT Read String.vi"("Name"=w298) -> ("String"=w297:string)  [unwired: 9 in, 1 out]
                n170 = Unbundle(w296) -> (w292:string[])
                n171 = Match First String(2:w292, 3:w297) -> (0:w293:i32)  [unwired: 1 out]
                n172 = property on="Ring" class="Ring (strict)"("Value"=w293, "Strings []"=w292) -> ()  [unwired: 2 in, 2 out]
                n173 = property on="Ring" class="Ring (strict)"("Visible"=TRUE) -> ()  [unwired: 2 in, 2 out]
                n174 = property on="Slider" class="Slide (strict)"("Visible"=FALSE) -> ()  [unwired: 2 in, 2 out]
              }
              frame "Color Enable  **" {
                n175 = Index Array(array=w304, index=4) -> (element=w305:cluster{string[]})
                n176 = call <vilib>:"NT Read String.vi"("Name"=w307) -> ("String"=w306:string)  [unwired: 9 in, 1 out]
                n177 = Unbundle(w305) -> (w301:string[])
                n178 = Match First String(2:w301, 3:w306) -> (0:w302:i32)  [unwired: 1 out]
                n179 = property on="Ring" class="Ring (strict)"("Value"=w302, "Strings []"=w301) -> ()  [unwired: 2 in, 2 out]
                n180 = property on="Ring" class="Ring (strict)"("Visible"=TRUE) -> ()  [unwired: 2 in, 2 out]
                n181 = property on="Slider" class="Slide (strict)"("Visible"=FALSE) -> ()  [unwired: 2 in, 2 out]
              }
              frame Default {
                n182 = property on="Ring" class="Ring (strict)"("Visible"=FALSE) -> ()  [unwired: 2 in, 2 out]
                n183 = property on="Slider" class="Slide (strict)"("Visible"=FALSE) -> ()  [unwired: 2 in, 2 out]
              }
              frame "Brightness  **", "Color Level  **", "Compression  **", "FPS  **", "Sharpness  **" {
                n184 = call <vilib>:"NT Read Number.vi"("Name"=w313) -> ("Numeric"=w312:dbl)  [unwired: 9 in, 1 out]
                n185 = local write "Slider"(w312) -> ()
                n186 = property on="Slider" class="Slide (strict)"("Visible"=TRUE, "Scale.Maximum"=100.0 ("Scale.Range:Maximum")) -> ()  [unwired: 2 in, 2 out]
                n187 = property on="Ring" class="Ring (strict)"("Visible"=FALSE) -> ()  [unwired: 2 in, 2 out]
              }
            }
          }
        }
        n188 = property on="Progress" class="Clust (strict)"("Visible"=FALSE) -> ()  [unwired: 2 in, 2 out]
      }
      event "Test Name": Mouse Enter {
        # "Populate the ring with the list of tests"
        n189 = event-data() -> ()  [unwired: 1 in, 1 out]
        n190 = call <vilib>:"NT Read String Array.vi"("Name"="TestMode/TestList") -> ("String Array"=w320:string[])  [unwired: 9 in, 1 out]
        n191 = Build Array (concatenate)("Select the test to run...", w320) -> (w319:string[])
        n192 = property on="Test Name" class="Ring (strict)"("Strings []"=w319) -> ()  [unwired: 2 in, 2 out]
      }
      event "Test Name": Value Change {
        w322 = FALSE ("Visible")
        # "Tell the robot the test name to run"
        n193 = event-data() -> ("NewVal"=w326:u16)  [unwired: 1 in]
        n194 = property on="Test Name" class="Ring (strict)"() -> ("Strings []"=w327:string[])  [unwired: 2 in, 2 out]
        n195 = local write "Progress"(T4 {"Test Progress"=0, "Test Progress Text"=""} ("Progress")) -> ()
        n196 = Index Array(array=w327, index=w326) -> (element=w325:string)
        n197 = call <vilib>:"NT Write String.vi"("String"=w325, "Name"="TestMode/TestName") -> ()  [unwired: 9 in, 1 out]
        n198 = property on="Progress" class="Clust (strict)"("Visible"=TRUE) -> ()  [unwired: 2 in, 2 out]
        n199 = property on="Motor" class="Clust (strict)"("Visible"=w322) -> ()  [unwired: 2 in, 2 out]
        n200 = property on="Slider" class="Slide (strict)"("Visible"=w322) -> ()  [unwired: 2 in, 2 out]
        n201 = property on="On/Off" class="Bool (strict)"("Visible"=w322) -> ()  [unwired: 2 in, 2 out]
        n202 = property on="Rev/Fwd" class="Clust (strict)"("Visible"=w322) -> ()  [unwired: 2 in, 2 out]
        n203 = property on="Ring" class="Ring (strict)"("Visible"=w322) -> ()  [unwired: 2 in, 2 out]
      }
      event "Listbox": Double Click {
        n204 = event-data() -> ("PlatMods.Shift"=w330:bool, "Row"=w332:i32)  [unwired: 1 in]
        n205 = case shown="False" w330 {
          tunnel: w332 -> [w336 _]
          tunnel: 1 -> [w335 _]
          frame False {
            n206 = property on="Listbox" class="LstBox (strict)"() -> ("Item Symbols"=w334:i32[])  [unwired: 2 in, 2 out]
            n207 = Replace Array Subset(array=w334, new element=w335, index=w336) -> (w333:i32[])
            n208 = property on="Listbox" class="LstBox (strict)"("Item Symbols"=w333) -> ()  [unwired: 2 in, 2 out]
          }
          frame True {
            w337 = 0 ("Top Row")
            n209 = property on="Listbox" class="LstBox (strict)"() -> ("Number of Rows"=w339:u32)  [unwired: 2 in, 2 out]
            n210 = Initialize Array(0, w339) -> (w338:i32[])
            n211 = property on="Listbox" class="LstBox (strict)"("Top Row"=w337, "Value"=w337, "Item Symbols"=w338) -> ()  [unwired: 2 in, 2 out]
          }
        }
      }
      event "Listbox": Key Down {
        n212 = event-data() -> ("VKey"=w343:T18)  [unwired: 1 in]
        n213 = case shown="\"Left\", \"Right\"" w343 {
          selector: w343 -> [w348 _]
          tunnel: eventvkey."Left" ("VKey") -> [w346 _]
          frame "Left", "Right" {
            n214 = Equal?(x=w346, y=w348) -> (x = y?=w347:bool)
            n215 = Select(t=0, s=w347, f=1) -> (s? t:f=w349:i32)
            n216 = property on="Listbox" class="LstBox (strict)"() -> ("Item Symbols"=w352:i32[])  [unwired: 2 in, 2 out]
            n217 = Replace Array Subset(array=w352, new element=w349, index="Listbox") -> (w351:i32[])
            n218 = property on="Listbox" class="LstBox (strict)"("Item Symbols"=w351) -> ()  [unwired: 2 in, 2 out]
          }
          frame Default {
          }
        }
      }
      event "DB Camera Config": Value Change {
        n219 = event-data() -> ("NewVal"=w356:bool)  [unwired: 1 in]
        n220 = case shown="False" w356 {
          tunnel: w355 -> [w365 _]
          tunnel: [w358 w376] -> w354
          tunnel: w353 -> [w357 w376]
          frame False {
            w372 = "Camera"
            w375 = FALSE ("Visible")
            n221 = local read "Camera Settings"() -> (w364:T1)
            n222 = Index Array(array=w365) -> (element=w368:cluster{string[]})  [unwired: 1 in]
            n223 = Unbundle(w364) -> ("Frate Rate"=w363:i32, "Compression"=w362:i32, "Size"=w366:u16)
            n224 = Unbundle(w368) -> (w367:string[])
            n225 = Index Array(array=w367, index=w366) -> (element=w361:string)
            n226 = call-poly <vilib>:"Write Key.vi"("section"=w372, "value"=w361, "key"="Size", "refnum"=w357) -> ("refnum out"=w374:T17)  [unwired: 2 in, 5 out]
            n227 = call-poly <vilib>:"Write Key.vi"("section"=w372, "value"=w363, "key"="FrameRate", "refnum"=w374) -> ("refnum out"=w373:T17)  [unwired: 1 in, 6 out]
            n228 = property on="Camera Settings" class="Clust (strict)"("Visible"=w375) -> ()  [unwired: 2 in, 2 out]
            n229 = local write "DB Camera Config"(w375) -> ()
            n230 = call-poly <vilib>:"Write Key.vi"("section"=w372, "value"=w362, "key"="Compression", "refnum"=w373) -> ("refnum out"=w359:T17)  [unwired: 1 in, 6 out]
            n231 = call <vilib>:"Close Config Data.vi"("refnum"=w359) -> ("file path"=w360:path)  [unwired: 2 in, 8 out]
            n232 = call <vilib>:"Open Config Data.vi"("configuration file path"=w360) -> ("refnum"=w358:T17)  [unwired: 8 in, 2 out]
          }
          frame True {
            n233 = property on="Camera Settings" class="Clust (strict)"("Visible"=TRUE) -> ()  [unwired: 2 in, 2 out]
          }
        }
      }
      event "Camera Settings": Value Change {
        n234 = event-data() -> ("NewVal"=w389:T1)  [unwired: 1 in]
        n235 = Index Array(array=w385) -> (element=w384:cluster{string[]})  [unwired: 1 in]
        n236 = Unbundle(w389) -> ("Frate Rate"=w380:i32, "Compression"=w379:i32, "Size"=w382:u16)
        n237 = Unbundle(w384) -> (w383:string[])
        n238 = Index Array(array=w383, index=w382) -> (element=w381:string)
        n239 = Format Into String(format string="%s   %dfps   %d%%", w381, w380, w379) -> (resulting string=w386:string)  [unwired: 2 in, 1 out]
        n240 = Build Array(w386) -> (w387:string[])
        n241 = property on="DB Camera Config" class="Bool (strict)"("Strings [4]"=w387) -> ()  [unwired: 2 in, 2 out]
      }
      event "Motor.Enable": Value Change {
        n242 = event-data() -> ("NewVal"=w395:bool)  [unwired: 1 in]
        n243 = Unbundle("Motor") -> ("Value"=w394:dbl)  [unwired: 1 out]
        n244 = Select(t=w394, s=w395, f=0.0) -> (s? t:f=w392:dbl)
        n245 = call <vilib>:"NT Write Number.vi"("Numeric"=w392, "Name"=w391) -> ()  [unwired: 9 in, 1 out]
      }
      event "Slider": Value Change {
        n246 = event-data() -> ("NewVal"=w398:dbl)  [unwired: 1 in]
        n247 = call <vilib>:"NT Write Number.vi"("Numeric"=w398, "Name"=w399) -> ()  [unwired: 9 in, 1 out]
      }
      event "On/Off": Value Change {
        n248 = event-data() -> ("NewVal"=w403:bool)  [unwired: 1 in]
        n249 = Boolean To (0,1)(Boolean=w403) -> (0, 1=w402:i16)
        n250 = call <vilib>:"NT Write Number.vi"("Numeric"=w402, "Name"=w401) -> ()  [unwired: 9 in, 1 out]
      }
      event "Rev/Fwd": Value Change {
        n251 = event-data() -> ("NewVal.Forward"=w411:bool, "NewVal.Reverse"=w410:bool)  [unwired: 1 in]
        n252 = Boolean To (0,1)(Boolean=w411) -> (0, 1=w407:i16)
        n253 = Boolean To (0,1)(Boolean=w410) -> (0, 1=w409:i16)
        n254 = Negate(x=w409) -> (-x=w408:i16)
        n255 = Add(x=w407, y=w408) -> (x+y=w406:i16)
        n256 = call <vilib>:"NT Write Number.vi"("Numeric"=w406, "Name"=w405) -> ()  [unwired: 9 in, 1 out]
      }
      event "Ring": Value Change {
        n257 = event-data() -> ("NewVal"=w415:u16)  [unwired: 1 in]
        n258 = property on="Ring" class="Ring (strict)"() -> ("Strings []"=w416:string[])  [unwired: 2 in, 2 out]
        n259 = Index Array(array=w416, index=w415) -> (element=w414:string)
        n260 = call <vilib>:"NT Write String.vi"("String"=w414, "Name"=w413) -> ()  [unwired: 9 in, 1 out]
      }
    }
  }
  n261 = Index Array(array=w15) -> (element=w16:cluster{string[]})  [unwired: 1 in]
  n262 = Unbundle(w16) -> (w14:string[])
  n263 = Match First String(2:w14, 3:w13) -> (0:w12:i32)  [unwired: 1 out]
  n264 = Bundle("value"=w18, "value"=w17, "index"=w12) -> (w6:cluster{"value":i32, "value":i32, "index":i32})  [unwired: 1 out]
  n265 = property on="On/Off" class="Bool (strict)"("Visible"=w29) -> ()  [unwired: 2 in, 2 out]
  n266 = property on="Motor" class="Clust (strict)"("Visible"=w29) -> ()  [unwired: 2 in, 2 out]
  n267 = property on="Progress" class="Clust (strict)"("Visible"=w29) -> ()  [unwired: 2 in, 2 out]
  n268 = property on="Ring" class="Ring (strict)"("Visible"=w29) -> ()  [unwired: 2 in, 2 out]
  n269 = property on="Camera Settings" class="Clust (strict)"("Val(Sgnl)"=w6) -> ()  [unwired: 2 in, 2 out]
  n270 = property on="Rev/Fwd" class="Clust (strict)"("Visible"=w29) -> ()  [unwired: 2 in, 2 out]
  n271 = property on="Camera Settings" class="Clust (strict)"("Visible"=w29) -> ()  [unwired: 2 in, 2 out]
  n272 = local write "DB Camera Config"(w29) -> ()
